vi "UI Gen Help Tags.vi"(8 "error in (no error)":errorcluster, 11 "Context":T1) -> (0 "error out":errorcluster)   [LabVIEW 2020, in "DocTool.lvlib"]
uses:
  DocTool.lvlib
  TDefs/Context.ctl
  Events/Events.ctl
  Events/UserEvent.ctl
  TDefs/State.ctl
  TDefs/States.ctl
  TDefs/Single File Properties.ctl
  TDefs/FP Items Properties.ctl
  TDefs/FP Item Properties.ctl
  TDefs/CopyTag.ctl
  StateMachine.lvlib
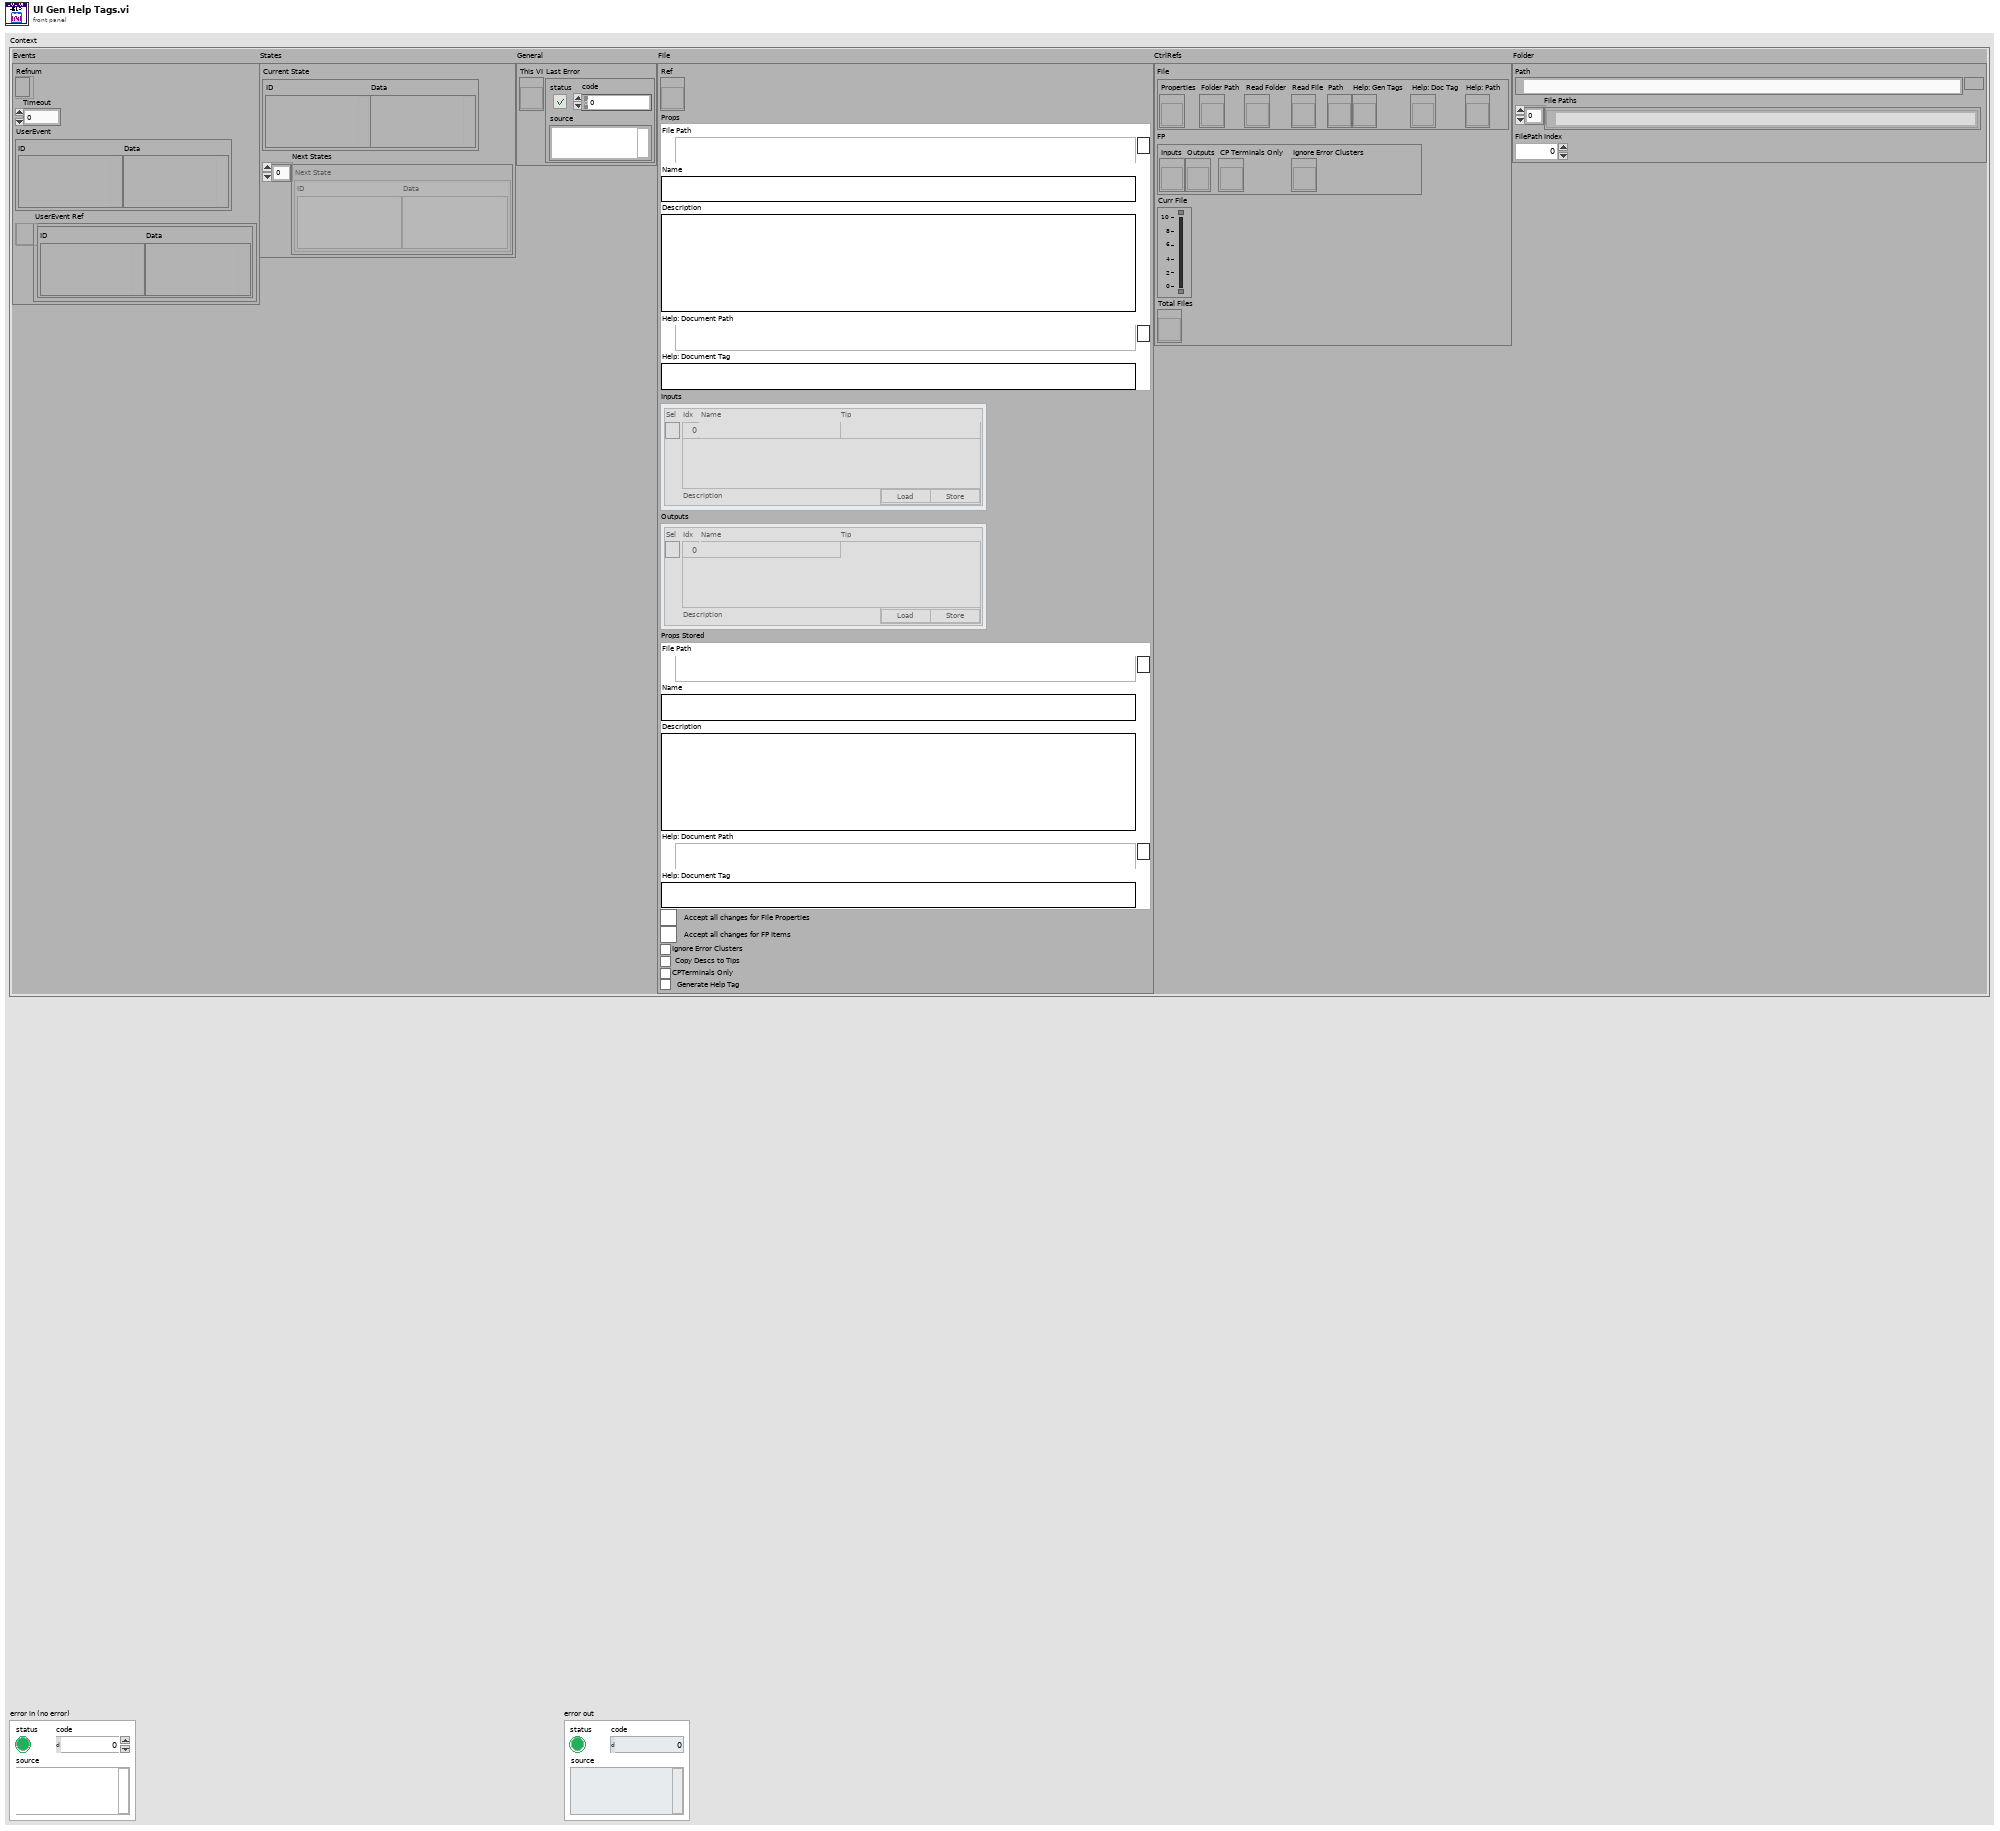
[diagram p1: front panel]
types:
  T1 = typedef "DocTool.lvlib/Context.ctl" = cluster{"Events":T2, "States":cluster{"Current State":T4, "Next States":T5}, "General":cluster{"This VI":refnum<vi>, "Last Error":errorcluster}, "File":cluster{"Ref":refnum<vi>, "Props":T6, "Inputs":T7, "Outputs":T7, "Props Stored":T6, "Write":bool, "Write FP":bool, "Ignore Error Clusters":bool, "Copy Descs to Tips":bool, "CPTerminals Only":bool, "Generate Help Tag":bool}, "CtrlRefs":cluster{"File":cluster{"Properties":refnum<vi>, "Folder Path":refnum<vi>, "Read Folder":refnum<vi>, "Read File":refnum<vi>, "Path":refnum<vi>, "Help: Gen Tags":refnum<vi>, "Help: Doc Tag":refnum<vi>, "Help: Path":refnum<vi>}, "FP":cluster{"Inputs":refnum<vi>, "Outputs":refnum<vi>, "CP Terminals Only":refnum<vi>, "Ignore Error Clusters":refnum<vi>}, "Curr File":refnum<vi>, "Total Files":refnum<vi>}, "Folder":cluster{"Path":path, "File Paths":path[], "FilePath Index":i32}}
  T2 = typedef "StateMachine.lvlib/Events.ctl" = cluster{"Refnum":refnum<event-registration>, "Timeout":i32, "UserEvent":T3, "UserEvent Ref":refnum<user-event>}
  T3 = typedef "StateMachine.lvlib/UserEvent.ctl" = cluster{"ID":variant, "Data":variant}
  T4 = typedef "StateMachine.lvlib/State.ctl" = cluster{"ID":variant, "Data":variant}
  T5 = typedef "StateMachine.lvlib/States.ctl" = T4[]
  T6 = typedef "DocTool.lvlib/Single File Properties.ctl" = cluster{"File Path":path, "Name":string, "Description":string, "Help: Document Path":path, "Help: Document Tag":string}
  T7 = typedef "DocTool.lvlib/FP Items Properties.ctl" = T8[]
  T8 = typedef "DocTool.lvlib/FP Item Properties.ctl" = cluster{"Sel":bool, "Idx":i32, "Name":string, "Description":string, "Tip":string, "Load Store":T9}
  T9 = typedef "DocTool.lvlib/CopyTag.ctl" = cluster{"Load":bool, "Store":bool}
  T10 = enum8{"Enabled", "Disabled", "Disabled and Grayed Out"}
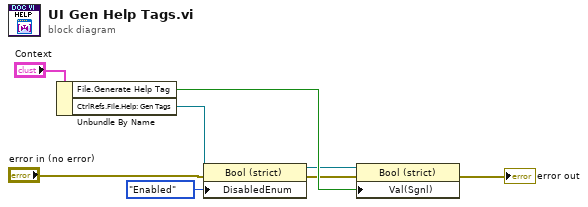
[diagram p0: block diagram]
diagram:
  n1 = Unbundle By Name("Context") -> ("File.Generate Help Tag"=w5:bool, "CtrlRefs.File.Help: Gen Tags"=w6:refnum<vi>)
  n2 = property class="Bool (strict)"(reference=w6, error in="error in (no error)", "DisabledEnum"=T10."Enabled" ("Disabled")) -> (reference out=w3:refnum<vi>, error out=w4:errorcluster)
  n3 = property class="Bool (strict)"(reference=w3, error in=w4, "Val(Sgnl)"=w5) -> (error out=→"error out":errorcluster)  [unwired: 1 out]
